vi "EnableDisable Control.vi"   [LabVIEW 2017, in "PXImc System Explorer.lvlib"]
uses:
  PXImc System Explorer.lvlib
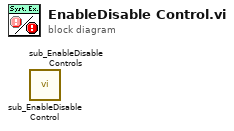
[diagram p0: block diagram]
diagram:
  n1 = call "sub_EnableDisable Control.vi"() -> ()  [unwired: 11 in, 1 out]
  n2 = call "sub_EnableDisable Controls.vi"() -> ()  [unwired: 11 in, 1 out]
